vi "Config End Pulse Event.vi"(6 "Input Event":string="0", 8 "error in":errorcluster, 9 "Channel (Channel A)":T1, 10 "Node In":string, 11 "VISA resource name":refnum<visa-resource-name>) -> (0 "error out":errorcluster, 2 "Node Out":string, 3 "VISA resource name out":refnum<visa-resource-name>, 4 "Command String":string)   [LabVIEW 2013, in "Keithley 2600 Series.lvlib"]
doc: "This VI configures the End Pulse even in the advanced trigger model.\n\n<b>Functions and Attributes Used</b>\nsmuX.trigger.endpulse.sequence.count\nsmuX.trigger.endpulse.sequence.number\nsmuX.trigger.endpulse.stimulus"
uses:
  Keithley 2600 Series.lvlib
  Private/GlobalVariables.vi
  Channel.ctl
panel:
  # "(c) 2008 Keithley Instruments, Inc.  ALL RIGHTS RESERVED."
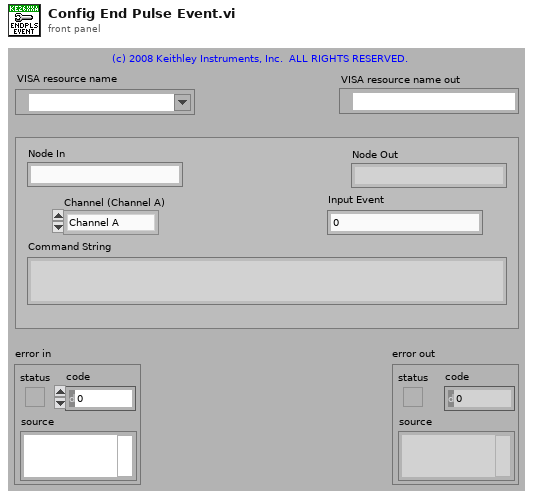
[diagram p1: front panel]
types:
  T1 = typedef "Keithley 2600 Series.lvlib/Channel.ctl" = enum32{"Channel A", "Channel B"}
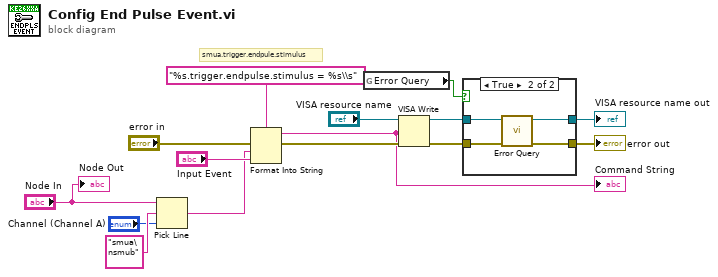
[diagram p0: block diagram]
diagram:
  # "smua.trigger.endpule.stimulus"
  n1 = Pick Line(string ("")="Node In", multi-line string="smua\nsmub", line index="Channel (Channel A)") -> (output string=w1:string)
  n2 = Format Into String(format string="%s.trigger.endpulse.stimulus = %s\\s", error in="error in", w1, "Input Event") -> (resulting string=w2:string, error out=w13:errorcluster)  [unwired: 1 in]
  "Command String" <- w2
  n3 = global read "GlobalVariables.vi" "Error Query"() -> (w12:bool)
  n4 = VISA Write(VISA resource name="VISA resource name", write buffer=w2, error in (no error)=w13) -> (VISA resource name out=w11:refnum<visa-resource-name>, error out=w10:errorcluster)  [unwired: 1 out]
  n5 = case shown="True" w12 {
    tunnel: w11 -> [w17 w21]
    tunnel: w10 -> [w16 w20]
    tunnel: [w17 w19] -> w4
    tunnel: [w16 w18] -> w3
    frame False {
    }
    frame True {
      n6 = call "Error Query.vi"("error in (no error)"=w20, "VISA resource name"=w21) -> ("error out"=w18:errorcluster, "VISA resource name out"=w19:refnum<visa-resource-name>)  [unwired: 8 out]
    }
  }
  "VISA resource name out" <- w4
  "error out" <- w3
  "Node Out" <- "Node In"
